vi "valve_only.vi"() -> ()   [LabVIEW 2019]
uses:
  Valve_class/Valve.lvclass
  ArduinoValve_class/ArduinoValve.lvclass
panel:
  in  "stop":bool
  in  "Pos 2":bool
  in  "Pos 1":bool
  in  "VISA resource name":refnum<visa-resource-name>
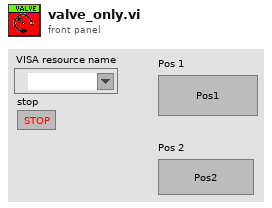
[diagram p1: front panel]
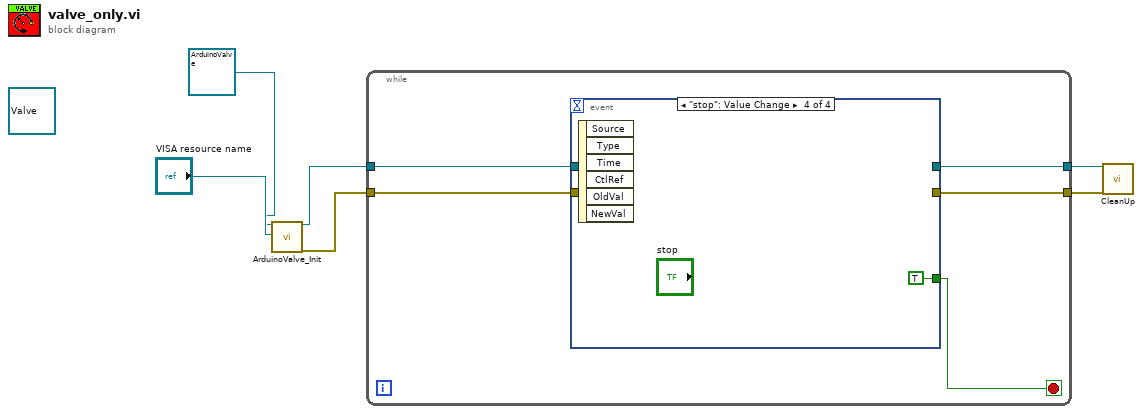
[diagram p0: block diagram]
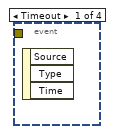
[diagram p2: hidden frame]
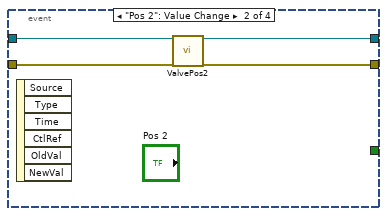
[diagram p3: hidden frame]
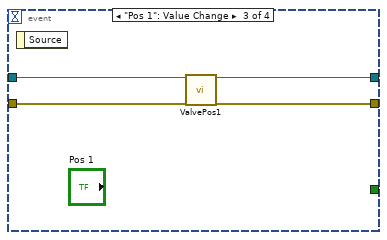
[diagram p4: hidden frame]
diagram:
  (unwired) refnum<class "Valve.lvclass"> refnum ("object in")
  n1 = call "ArduinoValve_Init.vi"("object in"=refnum<class "ArduinoValve.lvclass"> refnum ("ArduinoValve"), "VISA resource name"="VISA resource name") -> ("object out"=w4:refnum<class "ArduinoValve.lvclass">, "error out"=w1:errorcluster)  [unwired: 16 in]
  n2 = while {
    tunnel: w4 -> [w11]
    tunnel: w1 -> [w10]
    tunnel: [w9] -> w6
    tunnel: [w8] -> w5
    stop <- w7 stop-if-true
    n3 = event shown="[3] \"stop\": Value Change" {
      selector: _ -> [_ _ _ _]
      dyn-events: _ -> [_ _ _ _]
      timeout: _ -> [_ _ _ _]
      tunnel: w11 -> [_ w15 w19 _]
      tunnel: w10 -> [_ w14 w18 _]
      tunnel: [_ w13 w17 _] -> w9
      tunnel: [_ w12 w16 _] -> w8
      tunnel: [_ _ _ TRUE ("stop")] -> w7
      event Timeout {
        n4 = event-data() -> ()  [unwired: 1 in, 3 out]
      }
      event "Pos 2": Value Change {
        n5 = event-data() -> ()  [unwired: 1 in, 6 out]
        n6 = call-dynamic "ValvePos2.vi"("object in"=w15, "error in (no error)"=w14) -> ("object out"=w13:refnum<class "ArduinoValve.lvclass">, "error out"=w12:errorcluster)  [unwired: 16 in]
      }
      event "Pos 1": Value Change {
        n7 = event-data() -> ()  [unwired: 1 in, 1 out]
        n8 = call-dynamic "ValvePos1.vi"("object in"=w19, "error in (no error)"=w18) -> ("object out"=w17:refnum<class "ArduinoValve.lvclass">, "error out"=w16:errorcluster)  [unwired: 16 in]
      }
      event "stop": Value Change {
        n9 = event-data() -> ()  [unwired: 1 in, 6 out]
      }
    }
  }
  n10 = call-dynamic "CleanUp.vi"("object in"=w6, "error in (no error)"=w5) -> ()  [unwired: 16 in, 2 out]
